vi "23_2d.vi"() -> ()   [LabVIEW 2020]
uses:
  <vilib>/Analysis/1siggen.llb/Ramp Pattern by Delta.vi
  <vilib>/Analysis/NI_AALBase.lvlib
panel:
  out "Time":u32=401
  out "Start Array":i32[](array[numeric])
  out "product":u64=91408386135
  out "Array":u64[](array[numeric])=[351591, 259985]
  in  "Moves":i32=10000000
  in  "Cups":dbl=1000000.0 format="%#_13g"
  in  "Switch":bool
  in  "Input":string="925176834"
  in  "Input Test":string="389125467"
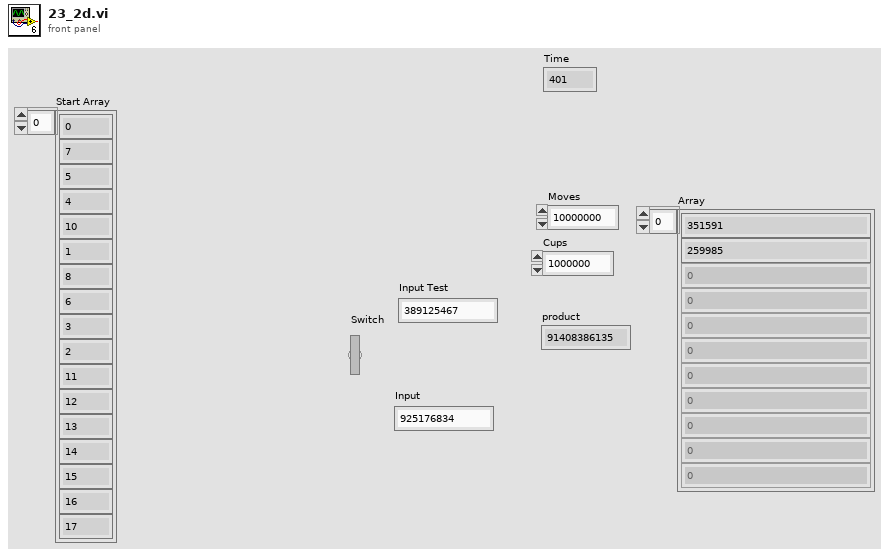
[diagram p1: front panel]
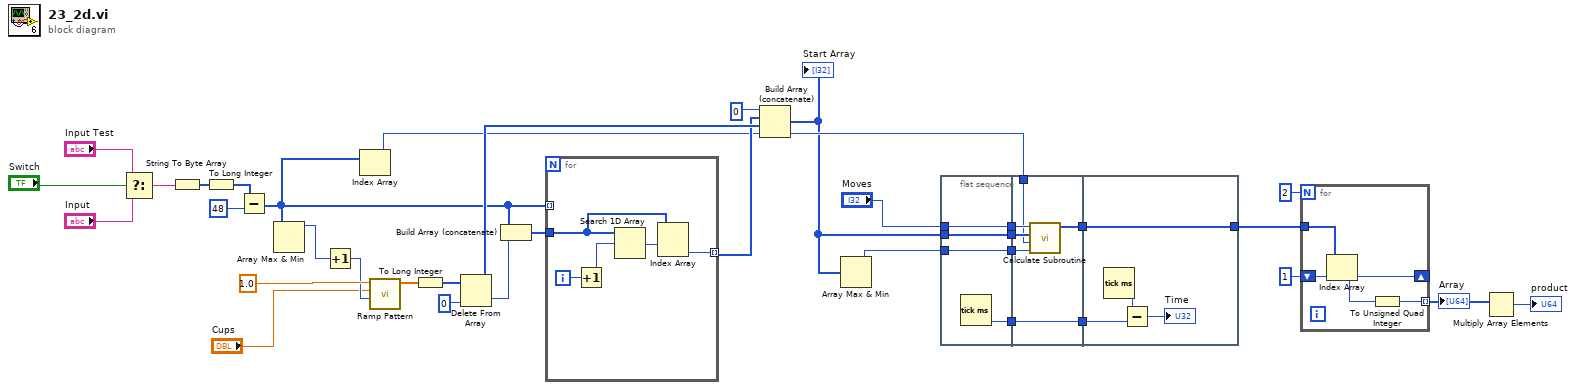
[diagram p0: block diagram]
diagram:
  n1 = Select(t="Input Test", s="Switch", f="Input") -> (s? t:f=w32:string)
  n2 = String To Byte Array(string=w32) -> (unsigned byte array=w31:u8[])
  n3 = To Long Integer(number=w31) -> (32bit integer=w29:i32[])
  n4 = Subtract(x=w29, y=48) -> (x-y=w13:i32[])
  n5 = Array Max & Min(array=w13) -> (max value=w25:i32)  [unwired: 3 out]
  n6 = Increment(x=w25) -> (x+1=w26:i32)
  n7 = Index Array(array=w13) -> (element=w4:i32)  [unwired: 1 in]
  n8 = call-poly <vilib>:"Ramp Pattern.vi"("start"=w26, "end"="Cups", "delta"=1.0) -> ("Ramp Pattern"=w27:dbl[])  [unwired: 6 in, 2 out]
  n9 = To Long Integer(number=w27) -> (32bit integer=w16:i32[])
  n10 = Delete From Array(array=w16, index=0) -> (deleted portion=w12:i32, array with subset deleted=w14:i32[])  [unwired: 1 in]
  n11 = Build Array (concatenate)(w13, w12) -> (w11:i32[])
  n12 = for {
    tunnel: w13 -> [_] mode=indexing
    tunnel: w11 -> [w38]
    tunnel: [w37] -> w10 mode=indexing
    i -> [w40]
    n13 = Increment(x=w40) -> (x+1=w39:i32)
    n14 = Search 1D Array(1D array=w38, element=w39) -> (index of element=w36:i32)  [unwired: 1 in]
    n15 = Index Array(array=w38, index #1=w36) -> (element #2=w37:i32)  [unwired: 1 in, 1 out]
  }
  n16 = Build Array (concatenate)(0, w10, w14, w4) -> (w3:i32[])
  "Start Array" <- w3
  n17 = Array Max & Min(array=w3) -> (max value=w2:i32)  [unwired: 3 out]
  n18 = flat-sequence {
    tunnel: w3 -> [w43]
    tunnel: "Moves" -> [w44]
    tunnel: [w44] -> w9
    tunnel: [w43] -> w8
    tunnel: [w42] -> w6
    tunnel: w2 -> [w41]
    tunnel: [w41] -> w1
    tunnel: w9 -> [w50]
    tunnel: w8 -> [w48]
    tunnel: [w49] -> w7
    tunnel: w6 -> [w47]
    tunnel: [w47] -> w5
    tunnel: w4 -> [w46]
    tunnel: w1 -> [w45]
    tunnel: [w54] -> w21
    tunnel: w7 -> [w54]
    tunnel: w5 -> [w52]
    frame #0 {
      n19 = Tick Count (ms)() -> (millisecond timer value=w42:u32)
    }
    frame #1 {
      n20 = call "Calculate Subroutine.vi"("Max Cup"=w45, "Start Cup"=w46, "Start Array"=w48, "Moves"=w50) -> ("End Array"=w49:i32[])  [unwired: 7 in]
    }
    frame #2 {
      n21 = Tick Count (ms)() -> (millisecond timer value=w53:u32)
      n22 = Subtract(x=w53, y=w52) -> (x-y=→"Time":u32)
    }
  }
  n23 = for {
    N: 2 -> [_]
    shift-right: [w56] -> _
    shift-left: 1 -> [w58]
    tunnel: [w55] -> w19 mode=indexing
    tunnel: w21 -> [w57]
    n24 = Index Array(array=w57, index=w58) -> (element=w56:i32)
    n25 = To Unsigned Quad Integer(1:w56) -> (0:w55:u64)
  }
  "Array" <- w19
  n26 = Multiply Array Elements(1:w19) -> (0:→"product":u64)
